vi "Generate Digital Output Signal.vi"(8 "error in":errorcluster, 11 "Data Cluster":T1={"Array"=[], "Boolean"=FALSE, "Engine Name"="", "Main Engine Response Q"=refnum, "TCP Engine Response Q"=refnum, "Varient Data"=variant(string ""), "Interupt Q"=refnum, "Start Notifier"=refnum, "Stop Notifier"=refnum, "DIO Configuration Cluster"={"Interface"="", "Interface Data"={"Command"="", "SubCmd"="", "Frequency"=0, "Data"=[]}}, "DO Task"="", "Command Q"=refnum, "DO Config Data"=[], "Log File Path"=path ""}) -> (0 "error out":errorcluster, 3 "Generation Stop":bool)   [LabVIEW 2024]
doc: "All Rights Reserved © 2017 SyncSols"
uses:
  Controls/Digital Output State Machine Data Cluster.ctl
  TCP Engine/Controls/TCP Engine I&O  Interupt Cluster.ctl
  Controls/DIO Configuration cluster.ctl
  Controls/DIO Interface Data.ctl
  Digital Dynamic Cluster.ctl
  Controls/DIO Commad Q Cluster.ctl
  Main Engine/Controls/Main Engine JSON Command State.ctl
  Host-DQMH/Configuration/DO Channel's.ctl
  TCP Engine/TCP Engine.lvlib
  Host-DQMH/Configuration/Configuration.lvlib
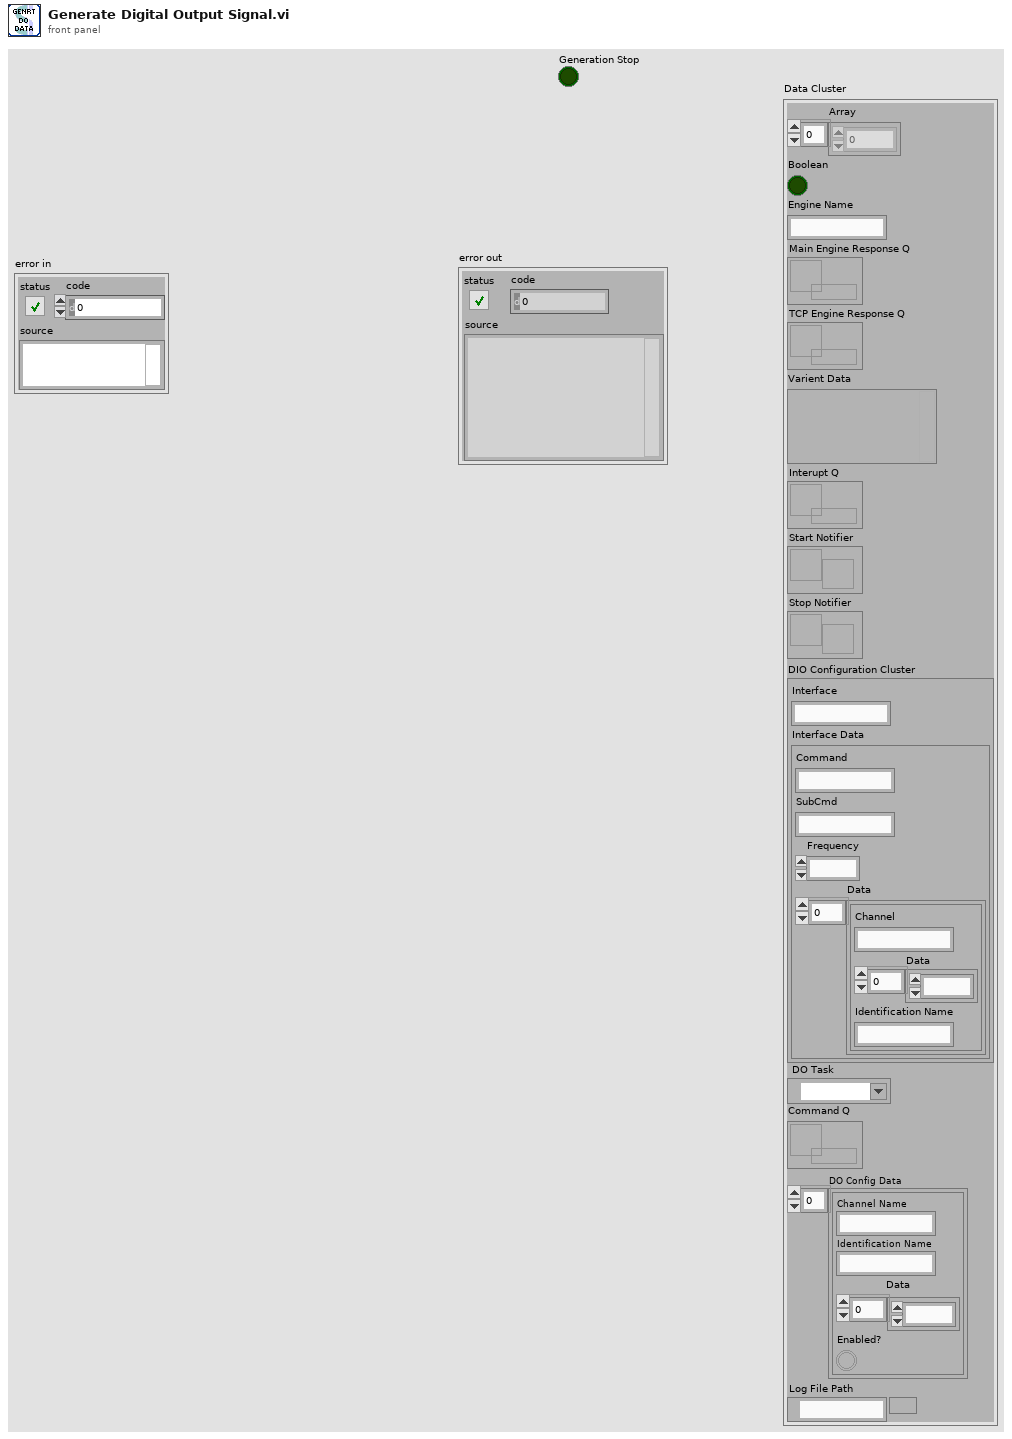
[diagram p1: front panel]
types:
  T1 = typedef "Digital Output State Machine Data Cluster.ctl" = cluster{"Array":dbl[], "Boolean":bool, "Engine Name":string, "Main Engine Response Q":refnum<queue>, "TCP Engine Response Q":refnum<queue>, "Varient Data":variant, "Interupt Q":refnum<queue>, "Start Notifier":refnum<notifier>, "Stop Notifier":refnum<notifier>, "DIO Configuration Cluster":T2, "DO Task":refnum<k21>, "Command Q":refnum<queue>, "DO Config Data":T5, "Log File Path":path}
  T2 = typedef "DIO Configuration cluster.ctl" = cluster{"Interface":string, "Interface Data":T3}
  T3 = typedef "DIO Interface Data.ctl" = cluster{"Command":string, "SubCmd":string, "Frequency":u16, "Data":T4[]}
  T4 = typedef "Digital Dynamic Cluster.ctl" = cluster{"Channel":string, "Data":u8[], "Identification Name":string}
  T5 = typedef "Configuration.lvlib/DO Channel's.ctl" = cluster{"Channel Name":string, "Identification Name":string, "Data":u8[], "Enabled?":bool}[]
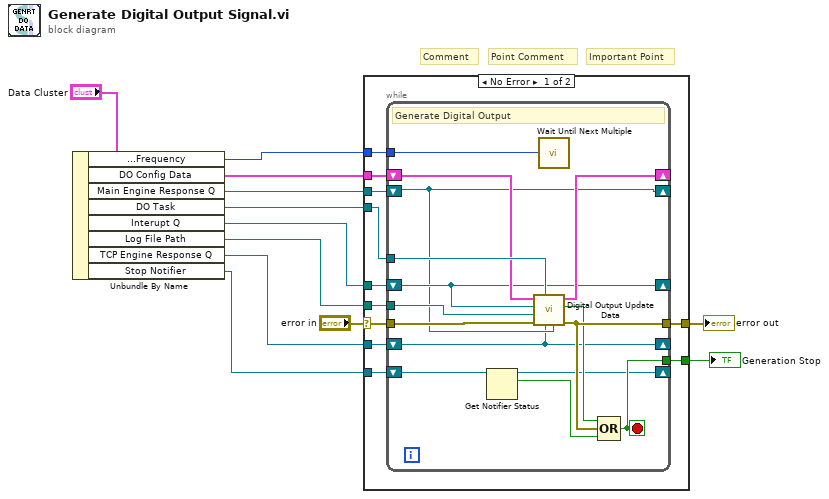
[diagram p0: block diagram]
diagram:
  # "Important Point"
  # "Point Comment"
  # "Comment"
  n1 = Unbundle By Name("Data Cluster") -> ("DIO Configuration Cluster.Interface Data.Frequency"=w8:u16, "DO Config Data"=w1:T5, "Main Engine Response Q"=w7:refnum<queue>, "DO Task"=w6:refnum<k21>, "Interupt Q"=w5:refnum<queue>, "Log File Path"=w4:path, "TCP Engine Response Q"=w3:refnum<queue>, "Stop Notifier"=w2:refnum<notifier>)
  n2 = case shown="No Error" "error in" {
    selector: "error in" -> [w20 w39]
    tunnel: [w19 w39] -> w12
    tunnel: w5 -> [w23 _]
    tunnel: w2 -> [w22 _]
    tunnel: w6 -> [w21 _]
    tunnel: w7 -> [w18 _]
    tunnel: w4 -> [w17 _]
    tunnel: w1 -> [w16 _]
    tunnel: [w15 _] -> w10
    tunnel: w8 -> [w14 _]
    tunnel: w3 -> [w13 _]
    frame No Error {
      n3 = while {
        tunnel: w21 -> [w36]
        tunnel: w20 -> [w35]
        tunnel: [w37] -> w19
        tunnel: w17 -> [w38]
        shift-right: [w34] -> _
        shift-left: w16 -> [w33]
        tunnel: [w31] -> w15
        tunnel: w14 -> [w30]
        shift-right: [w29] -> _
        shift-left: w23 -> [w29]
        shift-right: [w28] -> _
        shift-left: w18 -> [w28]
        shift-right: [w27] -> _
        shift-left: w13 -> [w27]
        shift-right: [w24] -> _
        shift-left: w22 -> [w26]
        stop <- w31 stop-if-true
        # "Generate Digital Output"
        n4 = Get Notifier Status(notifier=w26) -> (notifier out=w24:refnum<notifier>, current notification=w25:bool)  [unwired: 1 in, 3 out]
        n5 = call "Digital Output Update Data.vi"("Main Engine Response Q"=w28, "TCP Engine Response Q"=w27, "Task in"=w36, "error in"=w35, "Path"=w38, "Interupt Q"=w29, "DO Config Data"=w33) -> ("error out"=w37:errorcluster, "Stop"=w32:bool, "DO Config Data Out"=w34:T5)  [unwired: 2 in]
        n6 = call "Wait Until Next Multiple"("Count(mSec)"=w30) -> ()  [unwired: 1 out]
        n7 = Compound Arithmetic op=OR(w32, w37, w25) -> (w31:bool)
      }
    }
    frame Error {
    }
  }
  "error out" <- w12
  "Generation Stop" <- w10
